vi "camToStage_abs_3d.vi"(9 "transform cluster + actuator":T1, 11 "abs pixel location":dbl[](array[numeric])) -> (3 "pipette location (steps)":dbl[](array[numeric]))   [LabVIEW 2015]
uses:
  pipette cleaning/pressure box/cleaning_soft/controls/actuator_type.ctl
  pipette cleaning/pressure box/cleaning_soft/controls/actuator_cluster.ctl
  transform_properties_actuators.ctl
  controls/transform_cluster_actuator.ctl
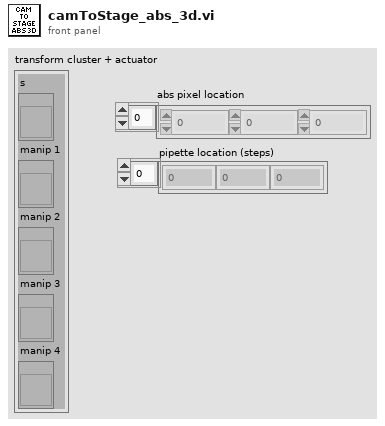
[diagram p1: front panel]
types:
  T1 = typedef "transform_cluster_actuator.ctl" = cluster{"s":refnum<vi>, "manip 1":refnum<vi>, "manip 2":refnum<vi>, "manip 3":refnum<vi>, "manip 4":refnum<vi>}
  T2 = typedef "transform_properties_actuators.ctl" = cluster{"theta (deg)":dbl, "X sc factor (px/step)":dbl, "Y sc factor (px/step)":dbl, "zero loc (x,y,z)":dbl[], "flip y?":bool, "flip x?":bool, "gamma (deg)":dbl, "flip z?":bool, "Z sc factor (px/step)":dbl, "actuator":T3, "safe space (steps)":i32[]}
  T3 = typedef "actuator_cluster.ctl" = cluster{"Actuator COM":refnum<visa-resource-name>, "Actuator type":T4}
  T4 = typedef "actuator_type.ctl" = enum16{"Scientifica", "Sutter", "Demo", "Off"}
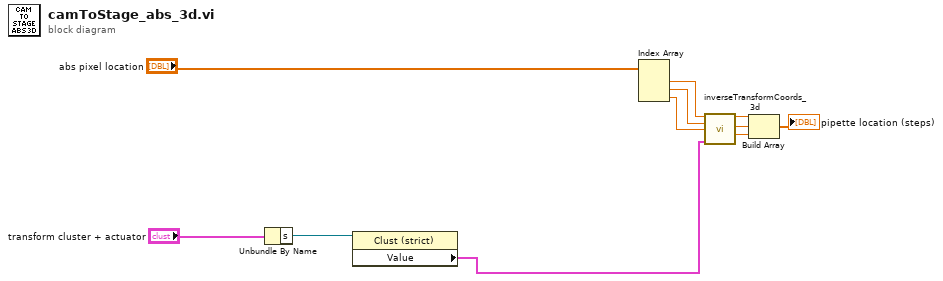
[diagram p0: block diagram]
diagram:
  n1 = Unbundle By Name("transform cluster + actuator") -> ("s"=w2:refnum<vi>)
  n2 = property class="Clust (strict)"(reference=w2) -> ("Value"=w1:T2)  [unwired: 1 in, 2 out]
  n3 = Index Array(array="abs pixel location") -> (element #1=w10:dbl, element #2=w9:dbl, element #3=w4:dbl)  [unwired: 3 in]
  n4 = call "inverseTransformCoords_3d.vi"("x"=w10, "y"=w9, "z"=w4, "transform properties"=w1) -> ("x out"=w8:dbl, "y out"=w7:dbl, "z out"=w3:dbl)  [unwired: 9 in]
  n5 = Build Array(w8, w7, w3) -> (→"pipette location (steps)":dbl[])
